vi "AnoopReadWriteVarsExample.vi"() -> ()   [LabVIEW 2020]
uses:
  <userlib>/Beckhoff-LabVIEW-Interface/_DependsOn/TypeDefs/Low-Levels/Symbol Interface Mode.ctl
panel:
  out "ReadGrpSymbols":string[](array[string])
  in  "stop":bool
  in  "FFTStatusUpdateFlags":T1
  in  "CalibrationResults":T2
  in  "WriteGrpSymbols 2":string[](array[string])=["192.168.0.20.1.1:851::GVL_LabviewDataShare.in_bAardvarkBoardError_labview", "192.168.0.20.1.1:851::GVL_LabviewDataShare.in_bAsic1CalibrationCompleted_labview", "192.168.0.20.1.1:851::GVL_LabviewDataShare.in_bAsic1CalibrationInProgress_labview", "192.168.0.20.1.1:851::GVL_LabviewDataShare.in_bAsic1CalibrationSuccess_labview", "192.168.0.20.1.1:851::GVL_LabviewDataShare.in_bAsic1FFTCompleted_labview", "192.168.0.20.1.1:851::GVL_LabviewDataShare.in_bAsic1FFTInProgress_labview", "192.168.0.20.1.1:851::GVL_LabviewDataShare.in_bAsic1FFTSuccess_labview", "192.168.0.20.1.1:851::GVL_LabviewDataShare.in_bAsic2CalibrationCompleted_labview", "192.168.0.20.1.1:851::GVL_LabviewDataShare.in_bAsic2CalibrationInProgress_labview", "192.168.0.20.1.1:851::GVL_LabviewDataShare.in_bAsic2CalibrationSuccess_labview", "192.168.0.20.1.1:851::GVL_LabviewDataShare.in_bAsic2FFTCompleted_labview", "192.168.0.20.1.1:851::GVL_LabviewDataShare.in_bAsic2FFTInProgress_labview", "192.168.0.20.1.1:851::GVL_LabviewDataShare.in_bAsic2FFTSuccess_labview", "192.168.0.20.1.1:851::GVL_LabviewDataShare.in_bCalResultsDBStoreSuccess_labview", "192.168.0.20.1.1:851::GVL_LabviewDataShare.in_bFFTResultsDBStoreSuccess_labview", "192.168.0.20.1.1:851::GVL_LabviewDataShare.in_bLabviewHandshakeBit", "192.168.0.20.1.1:851::GVL_LabviewDataShare.in_bLabviewResetComplete_labview", "192.168.0.20.1.1:851::GVL_LabviewDataShare.in_bLabviewResetSuccess_labview", "192.168.0.20.1.1:851::GVL_LabviewDataShare.in_bNIDaqError_labview", "192.168.0.20.1.1:851::GVL_LabviewDataShare.in_bPTC04BoardError_labview", "192.168.0.20.1.1:851::GVL_LabviewDataShare.in_bStartupInitializationCompleted_labview", "192.168.0.20.1.1:851::GVL_LabviewDataShare.in_bStartupInitializationSuccess_labview", "192.168.0.20.1.1:851::GVL_LabviewDataShare.in_strAsic1SerialNo_labview", "192.168.0.20.1.1:851::GVL_LabviewDataShare.in_strAsic2SerialNo_labview"]
  out "WriteGrpSymbols":string[](array[string])
  in  "EDP Hardware Reset Status":T3
  in  "EDP Startup Init Status":T4
  in  "SendHardwareResetStatus":bool
  in  "SendStartupInitStatus":bool
  in  "EDP Hardware Labview Error Status":T5
  in  "SendHardwareErrorStatus":bool
  in  "Symbol file path":path
  out "error out":errorcluster
  in  "error in (no error)":errorcluster
  out "BeckhoffParameters":T6
  in  "FFTResults":T7
  in  "CalibrationStatusUpdateFlags":T8
  in  "SendFFTResultsToBeckhoff":bool
  in  "SendCalResultsToBeckhoff":bool
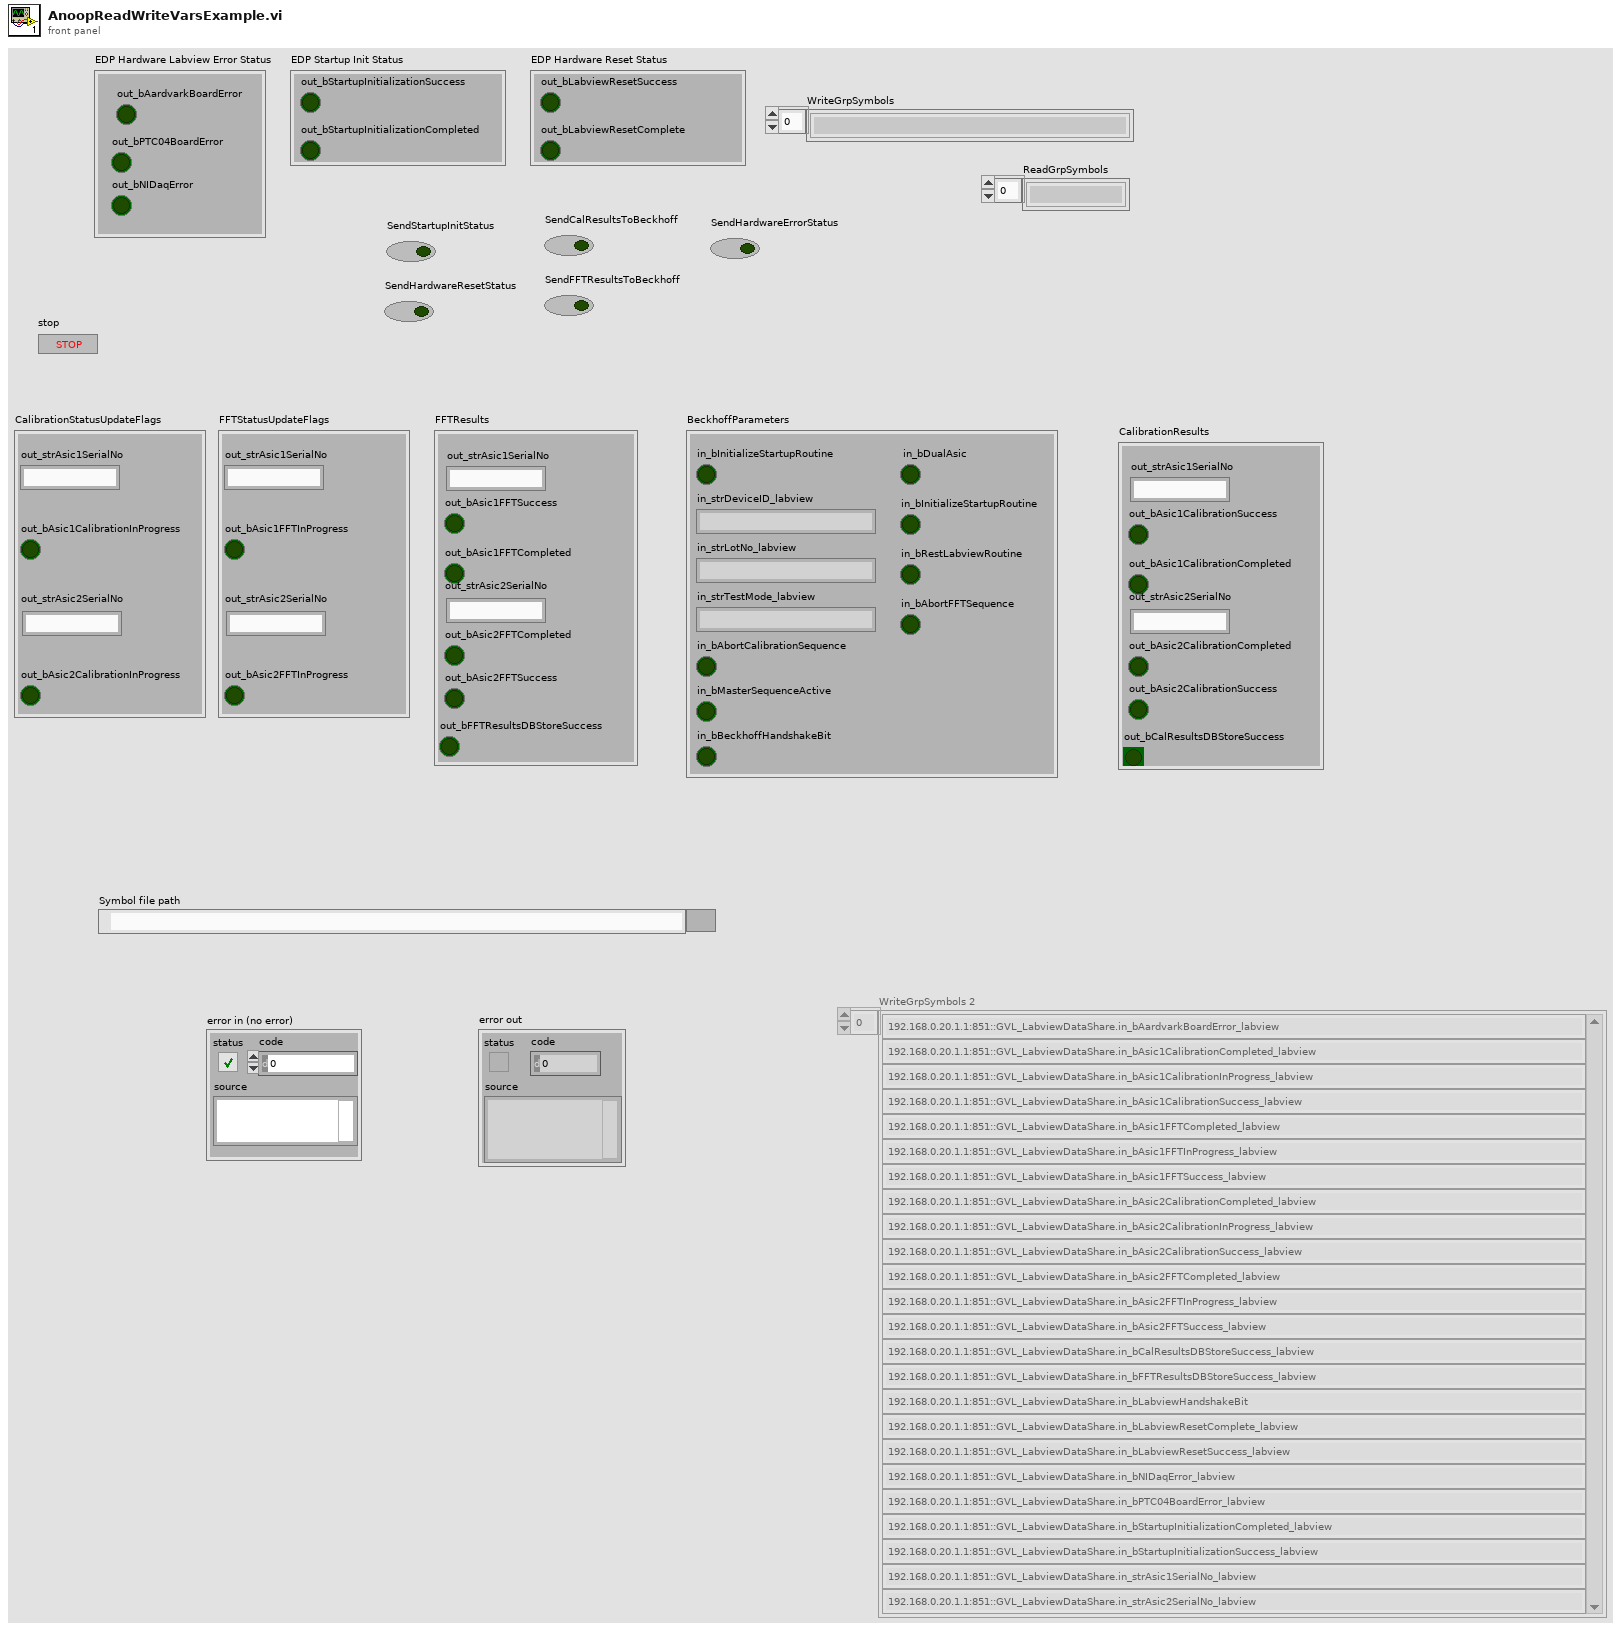
[diagram p1: front panel]
types:
  T1 = cluster{"out_strAsic1SerialNo":string, "out_bAsic1FFTInProgress":bool, "out_strAsic2SerialNo":string, "out_bAsic2FFTInProgress":bool}
  T2 = cluster{"out_strAsic1SerialNo":string, "out_bAsic1CalibrationSuccess":bool, "out_bAsic1CalibrationCompleted":bool, "out_strAsic2SerialNo":string, "out_bAsic2CalibrationCompleted":bool, "out_bCalResultsDBStoreSuccess":bool, "out_bAsic2CalibrationSuccess":bool}
  T3 = cluster{"out_bLabviewResetSuccess":bool, "out_bLabviewResetComplete":bool}
  T4 = cluster{"out_bStartupInitializationSuccess":bool, "out_bStartupInitializationCompleted":bool}
  T5 = cluster{"out_bAardvarkBoardError":bool, "out_bPTC04BoardError":bool, "out_bNIDaqError":bool}
  T6 = cluster{"in_bInitializeStartupRoutine":bool, "in_strDeviceID_labview":string, "in_strLotNo_labview":string, "in_strTestMode_labview":string, "in_bAbortCalibrationSequence":bool, "in_bMasterSequenceActive":bool, "in_bBeckhoffHandshakeBit":bool, "in_bDualAsic":bool, "in_bInitializeStartupRoutine":bool, "in_bRestLabviewRoutine":bool, "in_bAbortFFTSequence":bool}
  T7 = cluster{"out_strAsic1SerialNo":string, "out_bAsic1FFTSuccess":bool, "out_bAsic1FFTCompleted":bool, "out_strAsic2SerialNo":string, "out_bAsic2FFTCompleted":bool, "out_bFFTResultsDBStoreSuccess":bool, "out_bAsic2FFTSuccess":bool}
  T8 = cluster{"out_strAsic1SerialNo":string, "out_bAsic1CalibrationInProgress":bool, "out_strAsic2SerialNo":string, "out_bAsic2CalibrationInProgress":bool}
  T9 = typedef "Symbol Interface Mode.ctl" = enum16{"Read Only", "Write Only", "Read & Write"}
  T10 = cluster{"in_bInitializeStartupRoutine":bool, "in_strDeviceID_labview":string, "in_strLotNo_labview":string, "in_strTestMode_labview":string, "in_bAbortCalibrationSequence":bool, "in_bMasterSequenceActive":bool, "in_bBeckhoffHandshakeBit":bool, "in_bDualAsic":bool, "in_bInitializeStartupRoutine":bool, "in_bResetLabviewRoutine":bool, "in_bAbortFFTSequence":bool}
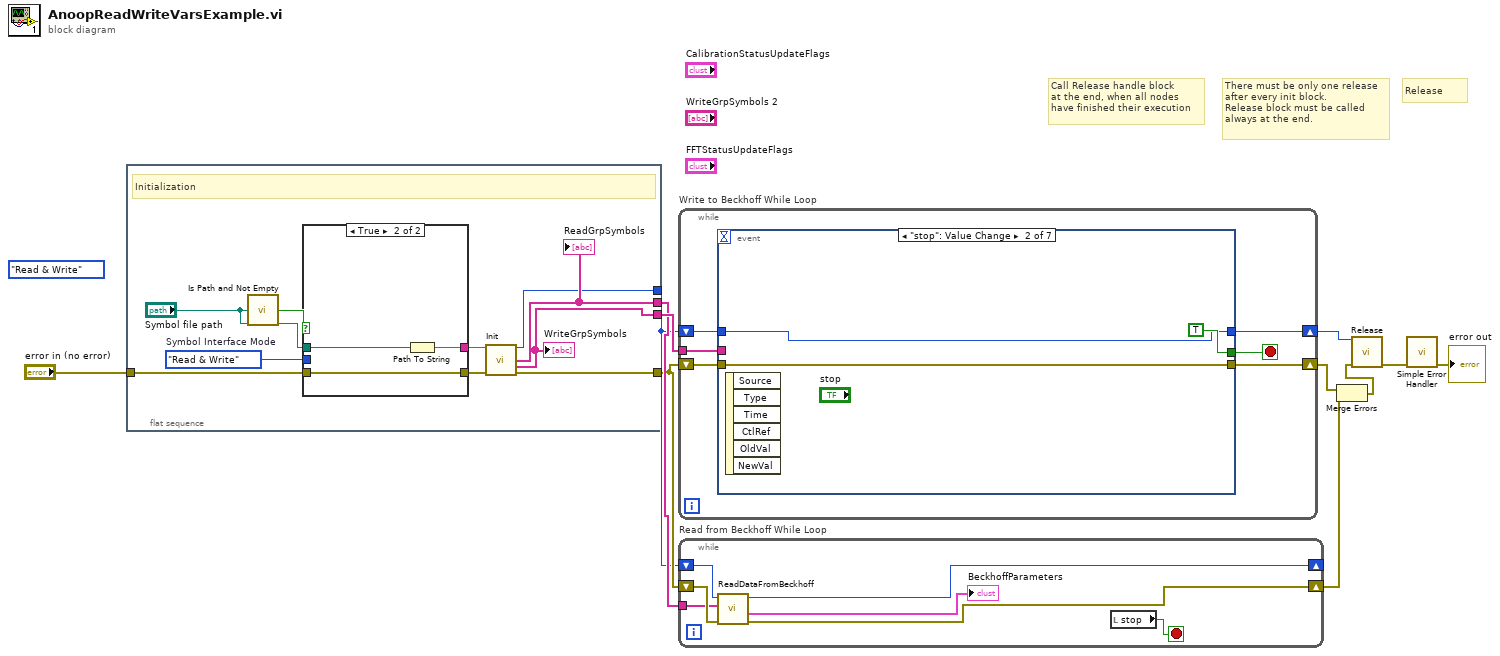
[diagram p0: block diagram]
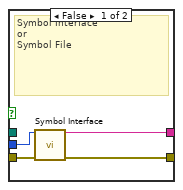
[diagram p2: hidden frame]
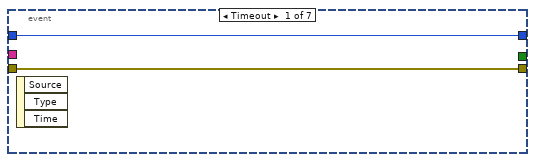
[diagram p3: hidden frame]
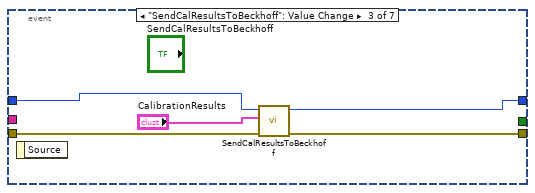
[diagram p4: hidden frame]
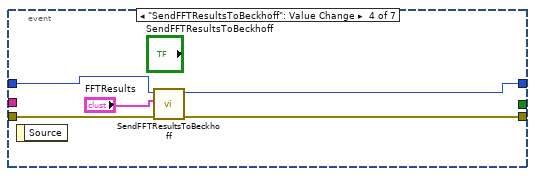
[diagram p5: hidden frame]
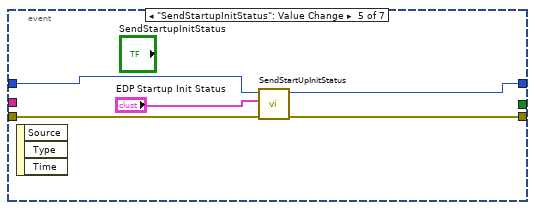
[diagram p6: hidden frame]
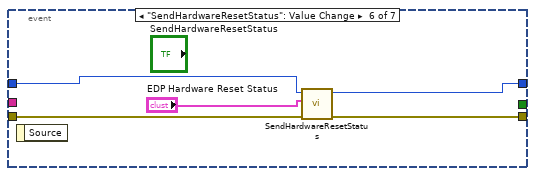
[diagram p7: hidden frame]
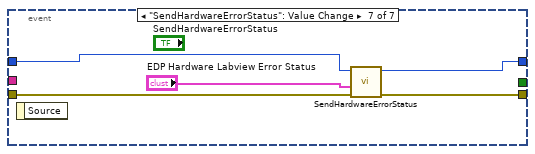
[diagram p8: hidden frame]
diagram:
  (unwired) Symbol_Interface_Mode."Read & Write" ("Symbol Interface Mode")
  # "Call Release handle block\nat the end, when all nodes\nhave finished their execution"
  # "There must be only one release\nafter every init block.\nRelease block must be called\nalways at the end."
  # "Release"
  n1 = flat-sequence {
    tunnel: "error in (no error)" -> [w16]
    tunnel: [w15] -> w8
    tunnel: [w14] -> w7
    tunnel: [w13] -> w6
    tunnel: [w12] -> w5
    frame #0 {
      w18 = Symbol_Interface_Mode."Read & Write"  # Symbol Interface Mode
      # "Initialization"
      n2 = call <vilib>:"Is Path and Not Empty.vi"("path"="Symbol file path") -> ("Is Path and Not Empty?"=w21:bool)  [unwired: 4 in]
      n3 = case shown="True" w21 {
        tunnel: [w25 w28] -> w17
        tunnel: "Symbol file path" -> [_ w27]
        tunnel: [w24 w26] -> w20
        tunnel: w18 -> [w23 _]
        tunnel: w16 -> [w22 w26]
        frame False {
          # "Symbol Interface\nor\nSymbol File"
          n4 = call <userlib>:"Symbol Interface.vi"("Symbol Interface Mode"=w23, "error in (no error)"=w22) -> ("PortInfo"=w25:string, "error out"=w24:errorcluster)  [unwired: 12 in]
        }
        frame True {
          n5 = Path To String(path=w27) -> (string=w28:string)
        }
      }
      n6 = call <userlib>:"Init.vi"("XMLDescription"=w17, "error in (no error)"=w20) -> ("Handle"=w12:u32, "ReadGrpSymbols"=w14:string[], "WriteGrpSymbols"=w15:string[], "error out"=w13:errorcluster)  [unwired: 9 in, 1 out]
      "WriteGrpSymbols" <- w15
      "ReadGrpSymbols" <- w14
    }
  }
  n7 = while "Write to Beckhoff While Loop" {
    shift-right: [w31] -> w10
    shift-left: w5 -> [w32]
    shift-right: [w33] -> w3
    shift-left: w6 -> [w34]
    tunnel: w8 -> [w30]
    stop <- w29 stop-if-true
    n8 = event shown="[1] \"stop\": Value Change" {
      selector: _ -> [_ _ _ _ _ _ _]
      dyn-events: _ -> [_ _ _ _ _ _ _]
      timeout: _ -> [_ _ _ _ _ _ _]
      tunnel: w34 -> [w36 w38 w43 w47 w54 w59 w64]
      tunnel: [w36 w38 w42 w46 w51 w58 w63] -> w33
      tunnel: w32 -> [w35 w37 w44 w49 w53 w57 w62]
      tunnel: [w35 w37 w41 w45 w52 w55 w61] -> w31
      tunnel: w30 -> [_ _ _ _ _ _ _]
      tunnel: [_ TRUE _ _ _ _ _] -> w29
      event Timeout {
        n9 = event-data() -> ()  [unwired: 1 in, 3 out]
      }
      event "stop": Value Change {
        n10 = event-data() -> ()  [unwired: 1 in, 6 out]
      }
      event "SendCalResultsToBeckhoff": Value Change {
        n11 = event-data() -> ()  [unwired: 1 in, 1 out]
        n12 = call "SendCalResultsToBeckhoff.vi"("error in (no error)"=w43, "CalResults"="CalibrationResults", "Handle In"=w44) -> ("error out"=w42:errorcluster, "Handle Out"=w41:u32)  [unwired: 7 in]
      }
      event "SendFFTResultsToBeckhoff": Value Change {
        n13 = event-data() -> ()  [unwired: 1 in, 1 out]
        n14 = call "SendFFTResultsToBeckhoff.vi"("error in (no error)"=w47, "FFTResults"="FFTResults", "Handle In"=w49) -> ("error out"=w46:errorcluster, "Handle Out"=w45:u32)  [unwired: 7 in]
      }
      event "SendStartupInitStatus": Value Change {
        n15 = event-data() -> ()  [unwired: 1 in, 3 out]
        n16 = call "SendStartUpInitStatus.vi"("error in (no error)"=w54, "EDP Startup Init Status"="EDP Startup Init Status", "Handle In"=w53) -> ("error out"=w51:errorcluster, "Handle Out"=w52:u32)  [unwired: 7 in]
      }
      event "SendHardwareResetStatus": Value Change {
        n17 = event-data() -> ()  [unwired: 1 in, 1 out]
        n18 = call "SendHardwareResetStatus.vi"("error in (no error)"=w59, "EDP Hardware Reset Status"="EDP Hardware Reset Status", "Handle In"=w57) -> ("error out"=w58:errorcluster, "Handle Out"=w55:u32)  [unwired: 7 in]
      }
      event "SendHardwareErrorStatus": Value Change {
        n19 = event-data() -> ()  [unwired: 1 in, 1 out]
        n20 = call "SendHardwareErrorStatus.vi"("error in (no error)"=w64, "EDP Hardware Labview Error Status"="EDP Hardware Labview Error Status", "Handle In"=w62) -> ("error out"=w63:errorcluster, "Handle Out"=w61:u32)  [unwired: 7 in]
      }
    }
  }
  n21 = while "Read from Beckhoff While Loop" {
    shift-right: [w69] -> _
    shift-left: w5 -> [w70]
    shift-right: [w68] -> w4
    shift-left: w6 -> [w71]
    tunnel: w7 -> [w66]
    stop <- w65 stop-if-true
    n22 = call "ReadDataFromBeckhoff.vi"("error in (no error)"=w71, "ReadGrpSymbols"=w66, "Handle In"=w70) -> ("error out"=w68:errorcluster, "BeckhoffParameters"=→"BeckhoffParameters":T10, "Handle Out"=w69:u32)  [unwired: 3 in, 1 out]
    n23 = local read "stop"() -> (w65:bool)
  }
  n24 = Merge Errors(w3, w4) -> (w2:errorcluster)
  n25 = call <userlib>:"Release.vi"("Handle"=w10, "error in (no error)"=w2) -> ("error out"=w1:errorcluster)  [unwired: 13 in]
  n26 = call <vilib>:"Simple Error Handler.vi"("error in (no error)"=w1) -> ("error out"=→"error out":errorcluster)  [unwired: 4 in, 4 out]
